vi "Load LUT from File.vi"(4 "error in (no error)":errorcluster, 7 "LUT File Path":path) -> (0 "error out":errorcluster, 3 "LUT Graph":cluster{dbl, dbl}[](array[cluster]))   [LabVIEW 2020]
panel:
  out "size(s)":i32
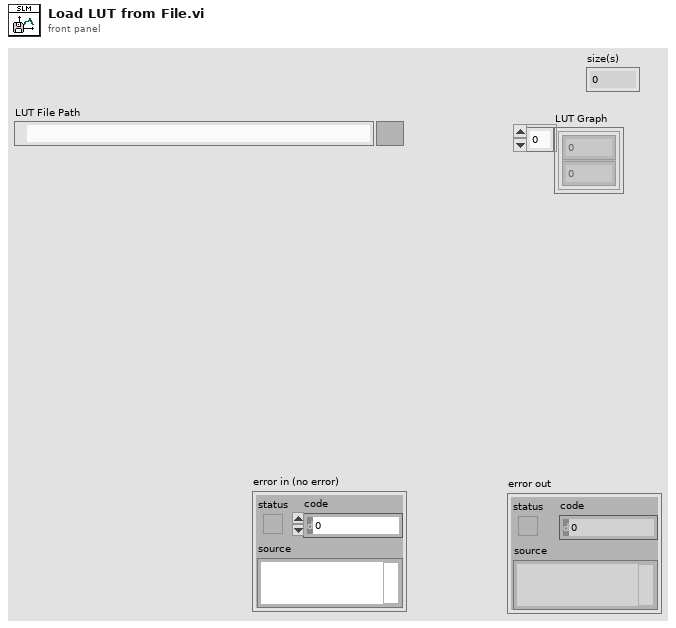
[diagram p1: front panel]
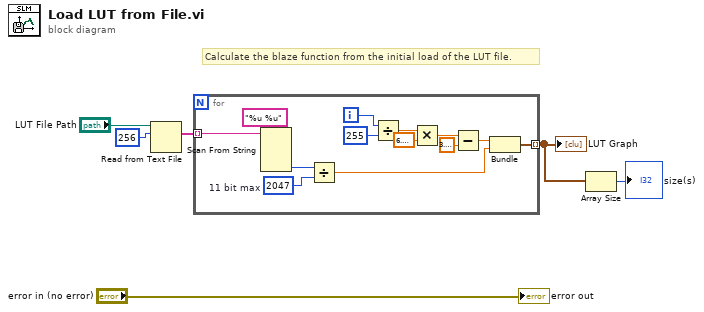
[diagram p0: block diagram]
diagram:
  # "Calculate the blaze function from the initial load of the LUT file."
  n1 = Read from Text File(file (use dialog)="LUT File Path", count=256) -> (text=w6:string[])  [unwired: 2 in, 3 out]
  n2 = for {
    tunnel: w6 -> [w19] mode=indexing
    tunnel: [w7] -> w2 mode=indexing
    i -> [w15]
    w16 = 2047  # 11 bit max
    n3 = Scan From String(format string="%u %u", input string=w19) -> (output 2=w17:u32)  [unwired: 5 in, 3 out]
    n4 = Divide(x=w17, y=w16) -> (x/y=w8:dbl)
    n5 = Divide(x=w15, y=255) -> (x/y=w10:dbl)
    n6 = Multiply(x=w10, y=6.283185307179586) -> (x*y=w12:dbl)
    n7 = Subtract(x=w12, y=3.141592653589793) -> (x-y=w9:dbl)
    n8 = Bundle(w9, w8) -> (w7:cluster{dbl, dbl})  [unwired: 1 out]
  }
  "LUT Graph" <- w2
  n9 = Array Size(array=w2) -> (size(s)=→"size(s)":i32)
  "error out" <- "error in (no error)"
